vi "Midbrain.vi"() -> ()   [LabVIEW 2012]
doc: "This VI acts as the MIDbrain in the Olin Robotics Architecture. It interacts with neural clusters on both the Forebrain and Hindbrain as shown in teh respective control panel dynamic documentation diagrams."
uses:
  <vilib>/Platform/TimedLoop/XDataNode/timing_clust.ctl
  <vilib>/Platform/TimedLoop/XDataNode/nitl_modes.ctl
  <vilib>/Platform/TimedLoop/XDataNode/wakeup.ctl
  GlobalHowAmI.vi
  GlobalACT.vi
  GlobalWhatAroundMe.vi
  GlobalWhereAmI.vi
  <vilib>/Platform/TimedLoop/XDataNode/XDataNode.xnode
  <vilib>/Platform/TimedLoop/XDataNode/XDNodeRunTimeDep.lvlib
panel:
  out "S-Wall Follow":dbl[](array[numeric])
  out "Lane Follow":dbl[](array[numeric])
  out "P-Wall Follow":dbl[](array[numeric])
  out "AvoidWall":dbl[](array[numeric])
  out "ObsAvoid":dbl[](array[numeric])
  out "ActCommand":dbl[](array[numeric])
  out "Act Command":cluster{"Velocity":dbl, "Direction":dbl}
  out "WhereAmI? Clean":T1
  out "HowAmI? Clean":cluster{"T":dbl, "Battery":dbl, "Temp":dbl}
  out "WhatAroundMe? Clean":cluster{"T":dbl, "Range":dbl, "Bearing":dbl}[](array[cluster])
  out "Cerr":bool
  out "Limbic":bool
  out "How?":bool
  out "Act":bool
  out "What?":bool
  in  "RT-stop":bool
  out "Where?":bool
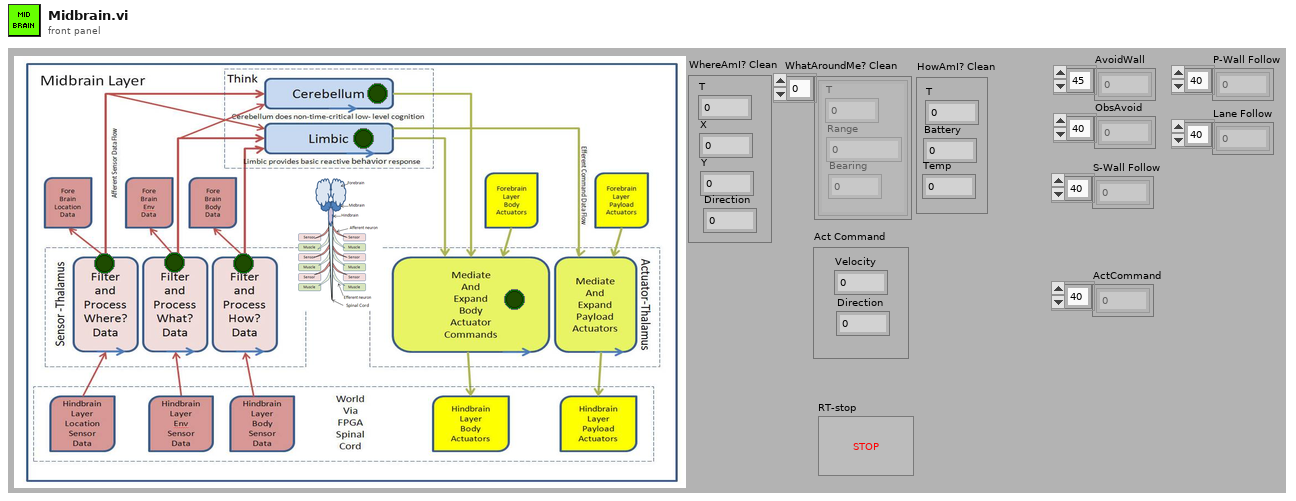
[diagram p1: front panel]
types:
  T1 = cluster{"T":dbl, "X":dbl, "Y":dbl, "Direction":dbl}
  T2 = typedef "XDNodeRunTimeDep.lvlib/timing_clust.ctl" = cluster{"Expected End [f-1]":u64, "Actual End [f-1]":u64, "Finished Late? [f-1]":bool, "Expected End [i-1]":u64, "Actual End [i-1]":u64, "Finished Late? [i-1]":bool, "Expected Start [i]":u64, "Actual Start [i]":u64, "Expected Start [f]":u64, "Actual Start [f]":u64, "Source Name":string, "Structure Name":string, "Period":i64, "Deadline":i64, "Offset":i64, "Start":i64, "Priority":i32, "Timeout":i32, "Mode":T3, "Wakeup Reason":T4, "Error":errorcluster, "Source Type":string, "Secondary Source Type":string, "Global End Time":u64, "Global Start Time":u64, "Frame Duration":u64, "Iteration Duration":u64, "Assigned CPU":i32, "I/O Scan Engine Mode":u32}
  T3 = typedef "XDNodeRunTimeDep.lvlib/nitl_modes.ctl" = enum32{"No Change", "Process missed periods, maintain original phase", "Discard missed periods, maintain original phase", "Process missed periods, ignore original phase", "Discard missed periods, ignore original phase"}
  T4 = typedef "XDNodeRunTimeDep.lvlib/wakeup.ctl" = enum32{"Normal", "Aborted", "Asynchronous wakeup", "Timing source error", "Timed loop error", "Timeout"}
  T5 = cluster{"VelCom":dbl, "BehCom":enum16{"OpenFieldTransit", "P-WallFollow", "S-WallFollow", "LaneFollow", "ManualMode"}}
  T6 = cluster{"AvoidWall":bool, "Wander":bool, "P-WallFollow":bool, "LaneFollow":bool, "S-WallFollow":bool}
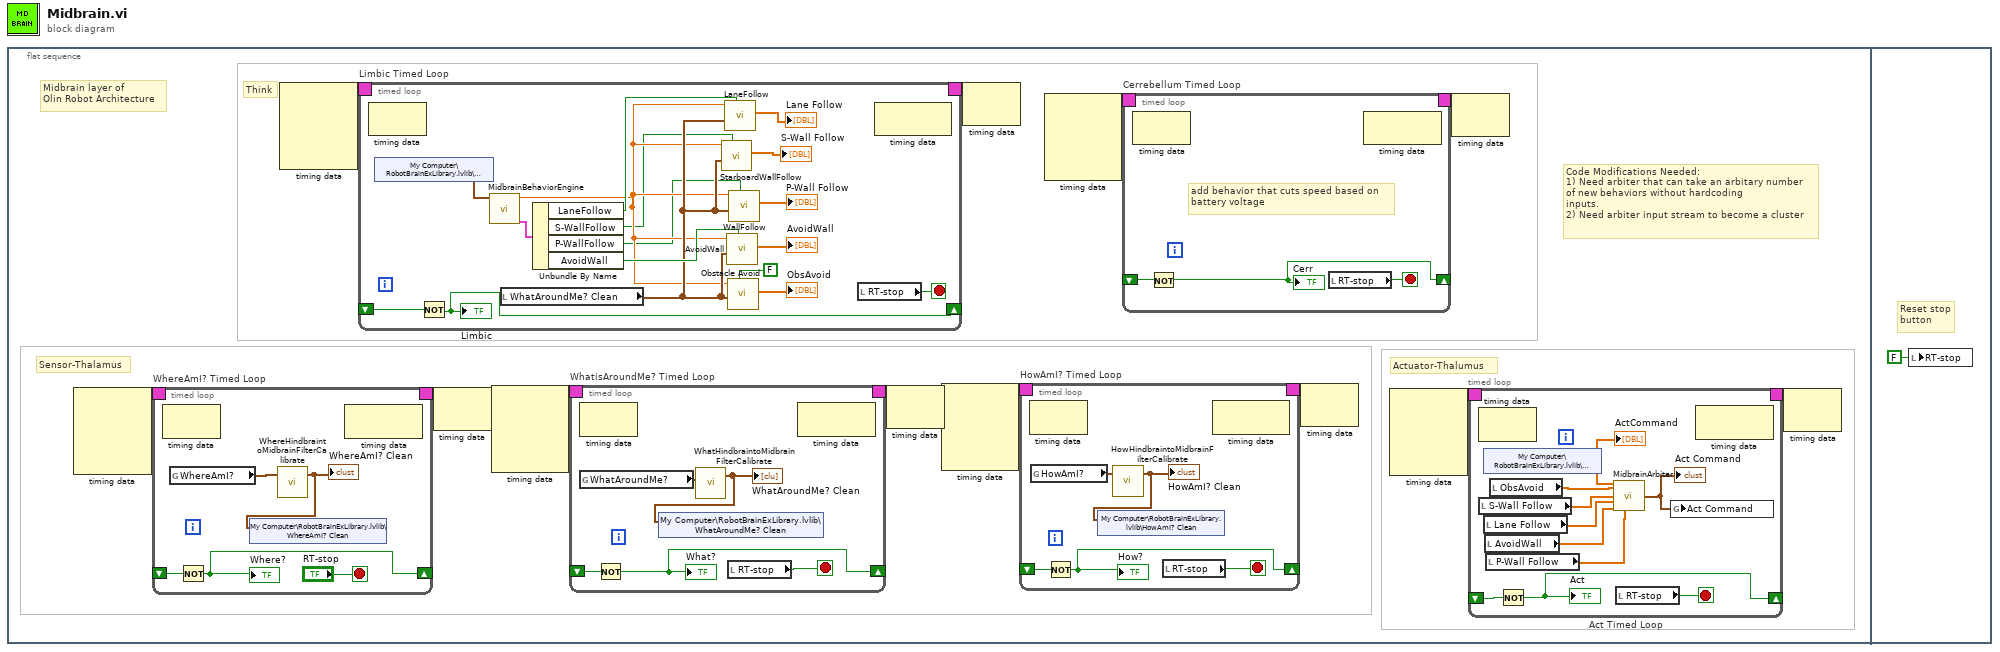
[diagram p0: block diagram]
diagram:
  n1 = flat-sequence {
    frame #0 {
      # "Code Modifications Needed:\n1) Need arbiter that can take an arbitary number\nof new behaviors without hardcoding \ninputs.\n2) Need arbiter input stream to become a cluster"
      # "Midbrain layer of\nOlin Robot Architecture"
      # "Think"
      # "Actuator-Thalumus"
      # "Sensor-Thalamus"
      n2 = node-c288 ("Input Node")() -> (w12:T2)  [unwired: 4 in]
      n3 = timed-loop "WhereAmI? Timed Loop" {
        timing: w12 -> [_]
        timing-out: [_] -> w11
        shift-right: [w76] -> _
        shift-left: _ -> [w77]
        stop <- "RT-stop" stop-if-true
        n4 = node-c288() -> ()  [unwired: 1 in, 1 out]
        n5 = global read "GlobalWhereAmI.vi" "WhereAmI?"() -> (w74:T1)
        n6 = Not(x=w77) -> (.not. x?=w76:bool)
        "Where?" <- w76
        n7 = call "WhereHindbraintoMidbrainFilterCalibrate.vi"("WhereAmI? Raw"=w74) -> ("WhereAmI? Clean"=w73:T1)  [unwired: 2 in]
        "WhereAmI? Clean" <- w73
        n8 = shared-variable "My Computer\\RobotBrainExLibrary.lvlib\\WhereAmI? Clean"(w73) -> ()  [unwired: 1 in, 1 out]
        n9 = node-c288() -> ()  [unwired: 1 in, 1 out]
      }
      n10 = node-c288 ("Input Node")() -> (w4:T2)  [unwired: 4 in]
      n11 = timed-loop "Limbic Timed Loop" {
        timing: w4 -> [_]
        timing-out: [_] -> w3
        shift-right: [w30] -> _
        shift-left: _ -> [w36]
        stop <- w35 stop-if-true
        n12 = node-c288() -> ()  [unwired: 1 in, 1 out]
        n13 = shared-variable "My Computer\\RobotBrainExLibrary.lvlib\\ForebrainCom"() -> (w22:T5)  [unwired: 1 in, 1 out]
        n14 = Not(x=w36) -> (.not. x?=w30:bool)
        "Limbic" <- w30
        n15 = call "MidbrainBehaviorEngine.vi"("ForebrainCom"=w22) -> ("BehaviorInhibit"=w29:T6, "VelCom"=w23:dbl)  [unwired: 9 in]
        n16 = local read "WhatAroundMe? Clean"() -> (w25:cluster{"T":dbl, "Range":dbl, "Bearing":dbl}[])
        n17 = Unbundle By Name(w29) -> ("LaneFollow"=w27:bool, "S-WallFollow"=w21:bool, "P-WallFollow"=w20:bool, "AvoidWall"=w28:bool)
        n18 = call "StarboardWallFollow.vi"("Inhibit"=w21, "WhatAroundMe? Clean"=w25, "Velocity"=w23) -> ("ActCommand"=→"S-Wall Follow":dbl[])  [unwired: 6 in, 2 out]
        n19 = call "LaneFollow.vi"("Inhibit"=w27, "WhatAroundMe? Clean"=w25, "Velocity"=w23) -> ("ActCommand"=→"Lane Follow":dbl[])  [unwired: 6 in, 2 out]
        n20 = call "AvoidWall.vi"("Inhibit"=w28, "WhatAroundMe? Clean"=w25, "Velocity"=w23) -> ("ActCommand"=→"AvoidWall":dbl[])  [unwired: 7 in, 1 out]
        n21 = call "Obstacle Avoid.vi"("Inhibit"=FALSE, "WhatAroundMe? Clean"=w25, "VelCom"=w23) -> ("ActCommand"=→"ObsAvoid":dbl[])  [unwired: 7 in, 1 out]
        n22 = call "WallFollow.vi"("Inhibit"=w20, "WhatAroundMe? Clean"=w25, "Velocity"=w23) -> ("ActCommand"=→"P-Wall Follow":dbl[])  [unwired: 6 in, 2 out]
        n23 = local read "RT-stop"() -> (w35:bool)
        n24 = node-c288() -> ()  [unwired: 1 in, 1 out]
      }
      n25 = node-c288(w11) -> ()  [unwired: 1 out]
      n26 = node-c288 ("Input Node")() -> (w10:T2)  [unwired: 4 in]
      n27 = timed-loop "WhatisAroundMe? Timed Loop" {
        timing: w10 -> [_]
        timing-out: [_] -> w9
        shift-right: [w67] -> _
        shift-left: _ -> [w68]
        stop <- w66 stop-if-true
        n28 = node-c288() -> ()  [unwired: 1 in, 1 out]
        n29 = global read "GlobalWhatAroundMe.vi" "WhatAroundMe?"() -> (w65:cluster{"T":dbl, "Range":dbl, "Bearing":dbl}[])
        n30 = Not(x=w68) -> (.not. x?=w67:bool)
        "What?" <- w67
        n31 = call "WhatHindbraintoMidbrainFilterCalibrate.vi"("WhatAroundMe?"=w65) -> ("WhatAroundMe? Clean"=w64:cluster{"T":dbl, "Range":dbl, "Bearing":dbl}[])  [unwired: 2 in]
        "WhatAroundMe? Clean" <- w64
        n32 = shared-variable "My Computer\\RobotBrainExLibrary.lvlib\\WhatAroundMe? Clean"(w64) -> ()  [unwired: 1 in, 1 out]
        n33 = local read "RT-stop"() -> (w66:bool)
        n34 = node-c288() -> ()  [unwired: 1 in, 1 out]
      }
      n35 = node-c288(w9) -> ()  [unwired: 1 out]
      n36 = node-c288 ("Input Node")() -> (w6:T2)  [unwired: 4 in]
      n37 = node-c288(w3) -> ()  [unwired: 1 out]
      n38 = timed-loop "HowAmI? Timed Loop" {
        timing: w6 -> [_]
        timing-out: [_] -> w5
        shift-right: [w41] -> _
        shift-left: _ -> [w45]
        stop <- w44 stop-if-true
        n39 = node-c288() -> ()  [unwired: 1 in, 1 out]
        n40 = global read "GlobalHowAmI.vi" "HowAmI?"() -> (w43:cluster{"T":dbl, "Battery":dbl, "Temp":dbl})
        n41 = Not(x=w45) -> (.not. x?=w41:bool)
        "How?" <- w41
        n42 = call "HowHindbraintoMidbrainFilterCalibrate.vi"("HowAmI?"=w43) -> ("HowAmI? Clean"=w42:cluster{"T":dbl, "Battery":dbl, "Temp":dbl})  [unwired: 2 in]
        "HowAmI? Clean" <- w42
        n43 = shared-variable "My Computer\\RobotBrainExLibrary.lvlib\\HowAmI? Clean"(w42) -> ()  [unwired: 1 in, 1 out]
        n44 = local read "RT-stop"() -> (w44:bool)
        n45 = node-c288() -> ()  [unwired: 1 in, 1 out]
      }
      n46 = node-c288 ("Input Node")() -> (w2:T2)  [unwired: 4 in]
      n47 = timed-loop "Cerrebellum Timed Loop" {
        timing: w2 -> [_]
        timing-out: [_] -> w1
        shift-right: [w14] -> _
        shift-left: _ -> [w15]
        stop <- w13 stop-if-true
        # "add behavior that cuts speed based on \nbattery voltage"
        n48 = node-c288() -> ()  [unwired: 1 in, 1 out]
        n49 = Not(x=w15) -> (.not. x?=w14:bool)
        "Cerr" <- w14
        n50 = local read "RT-stop"() -> (w13:bool)
        n51 = node-c288() -> ()  [unwired: 1 in, 1 out]
      }
      n52 = node-c288(w5) -> ()  [unwired: 1 out]
      n53 = node-c288 ("Input Node")() -> (w8:T2)  [unwired: 4 in]
      n54 = node-c288(w1) -> ()  [unwired: 1 out]
      n55 = timed-loop "Act Timed Loop" {
        timing: w8 -> [_]
        timing-out: [_] -> w7
        shift-right: [w58] -> _
        shift-left: _ -> [w59]
        stop <- w57 stop-if-true
        n56 = node-c288() -> ()  [unwired: 1 in, 1 out]
        n57 = local read "S-Wall Follow"() -> (w52:dbl[])
        n58 = shared-variable "My Computer\\RobotBrainExLibrary.lvlib\\ActCommand"() -> (w55:dbl[])  [unwired: 1 in, 1 out]
        "ActCommand" <- w55
        n59 = local read "Lane Follow"() -> (w51:dbl[])
        n60 = local read "AvoidWall"() -> (w53:dbl[])
        n61 = local read "P-Wall Follow"() -> (w50:dbl[])
        n62 = local read "ObsAvoid"() -> (w54:dbl[])
        n63 = Not(x=w59) -> (.not. x?=w58:bool)
        "Act" <- w58
        n64 = call "MidbrainArbiter.vi"("ForebrainInput"=w55, "ObstacleAvoid"=w54, "S-Wall Follow"=w52, "Lane Follow"=w51, "Wall Avoid"=w53, "P-Wall Follow"=w50) -> ("Act Command"=w56:cluster{"Velocity":dbl, "Direction":dbl})  [unwired: 9 in]
        "Act Command" <- w56
        n65 = local read "RT-stop"() -> (w57:bool)
        n66 = global write "GlobalACT.vi" "Act Command"(w56) -> ()
        n67 = node-c288() -> ()  [unwired: 1 in, 1 out]
      }
      n68 = node-c288(w7) -> ()  [unwired: 1 out]
    }
    frame #1 {
      # "Reset stop\nbutton"
      n69 = local write "RT-stop"(FALSE ("RT-stop")) -> ()
    }
  }
